vi "NI 9260 Generate Signal (Host).vi"() -> ()   [LabVIEW 2021]
uses:
  <vilib>/LabVIEW Targets/FPGA/cRIO/shared/nicrio_ModuleControls/nicrio_cRIO-9260_DataRatesRing2.ctl
  <vilib>/FPGAPlugInAG/cRIO-9053/niLvFpga_Open_cRIO-9053.vi
  <vilib>/rvi/interface/common/dynamic/niFpgaDynamicAddResources.vi
  <vilib>/Utility/error.llb/Error Cluster From Error Code.vi
  <vilib>/rvi/errors/niLvFpgaAdjustHostInterfaceError.vi
  <vilib>/rvi/interface/common/niFpgaWaitOnOcc.vi
  <vilib>/FPGAPlugInAG/Dynamic/niLvFpga_Run_Dynamic.vi
  <vilib>/FPGAPlugInAG/Dynamic/niLvFpga_Close_Dynamic.vi
  <vilib>/rvi/interface/nirviOpenFPGA/nirviOpenFPGA.xnode
  FPGA Bitfiles/crio-ni9260_FPGATarget_NI9260GenerateSi_CtzEkzqCx3U.lvbitx
  NI 9260 Generate Signal (FPGA).vi
  <vilib>/rvi/interface/nirviReadWriteControl/nirviReadWriteControl.xnode
  <vilib>/rvi/interface/nirviMethod/nirviMethod.xnode
  <vilib>/rvi/interface/nirviCloseFPGA/nirviCloseFPGA.xnode
  <vilib>/rvi/interface/Simulation/niFpgaSimulationCallBeginRW.vi
  <vilib>/FPGAPlugInAG/Dynamic/niLvFpga_WriteFifo_Dynamic.vi
  <vilib>/rvi/errors/niLvFpgaMergeErrorWithErrorCode.vi
  NiFpgaLv.dll
  <vilib>/FPGAPlugInAG/Dynamic/niLvFpga_ConfigureFifo_Dynamic.vi
panel:
  out "loop time (ms)":u32
  in  "Waveform":T1(ring)=enum."Square Wave"
  in  "Host Loop Rate (ms)":u32=100
  out "FIFO Time Out":bool
  out "Overvoltage":bool[](array[boolean])
  out "Underflow":bool[](array[boolean])
  in  "Sine Waveform Settings":T2(array[cluster])=[{"Frequency (Hz)"=1000.0, "Amplitude (V)"=4.0, "Offset (V)"=0.0, "Phase (deg)"=0.0}, {"Frequency (Hz)"=100.0, "Amplitude (V)"=3.0, "Offset (V)"=0.0, "Phase (deg)"=0.0}]
  in  "stop":bool
  out "FPGA Error out":errorcluster
  in  "Number of Samples per channel":dbl=51200.0 format="%.2p"
  out "Analog Output":waveform(dbl)[](graph)
  in  "Data Rate":T3=1 items=["51.200 kS/s (NI 9260)"=1, "25.600 kS/s (NI 9260)"=2, "17.067 kS/s (NI 9260)"=3, "12.800 kS/s (NI 9260)"=4, "10.240 kS/s (NI 9260)"=5, "8.533 kS/s (NI 9260)"=6, "7.314 kS/s (NI 9260)"=7, "6.400 kS/s (NI 9260)"=8, "5.689 kS/s (NI 9260)"=9, "5.120 kS/s (NI 9260)"=10, "4.654 kS/s (NI 9260)"=11, "4.267 kS/s (NI 9260)"=12, "3.938 kS/s (NI 9260)"=13, "3.657 kS/s (NI 9260)"=14, "3.413 kS/s (NI 9260)"=15, "3.200 kS/s (NI 9260)"=16, "3.012 kS/s (NI 9260)"=17, "2.845 kS/s (NI 9260)"=18, "2.695 kS/s (NI 9260)"=19, "2.560 kS/s (NI 9260)"=20, "2.438 kS/s (NI 9260)"=21, "2.328 kS/s (NI 9260)"=22, "2.226 kS/s (NI 9260)"=23, "2.133 kS/s (NI 9260)"=24, "2.048 kS/s (NI 9260)"=25, "1.969 kS/s (NI 9260)"=26, "1.896 kS/s (NI 9260)"=27, "1.829 kS/s (NI 9260)"=28, "1.765 kS/s (NI 9260)"=29, "1.707 kS/s (NI 9260)"=30, "1.652 kS/s (NI 9260)"=31]
  out "Host Error out":errorcluster
  # "Overview: Demonstrates how to generate a sine wave from the NI 9260\nRequirements: LabVIEW Full Development System, LV FPGA, and NI RIO\nInstructions: \n1. The NI 9260 will drive its outputs to 0 volts when the module receives a start command. Some DUTs will be affected by the sudden drop to zero from the previous value seen at the output. See the  NI 9260 Advanced example for how to mitigate this behavior.  \n2. Run this VI."
  # "CH0"
  # "CH1"
  # "CH0"
  # "CH1"
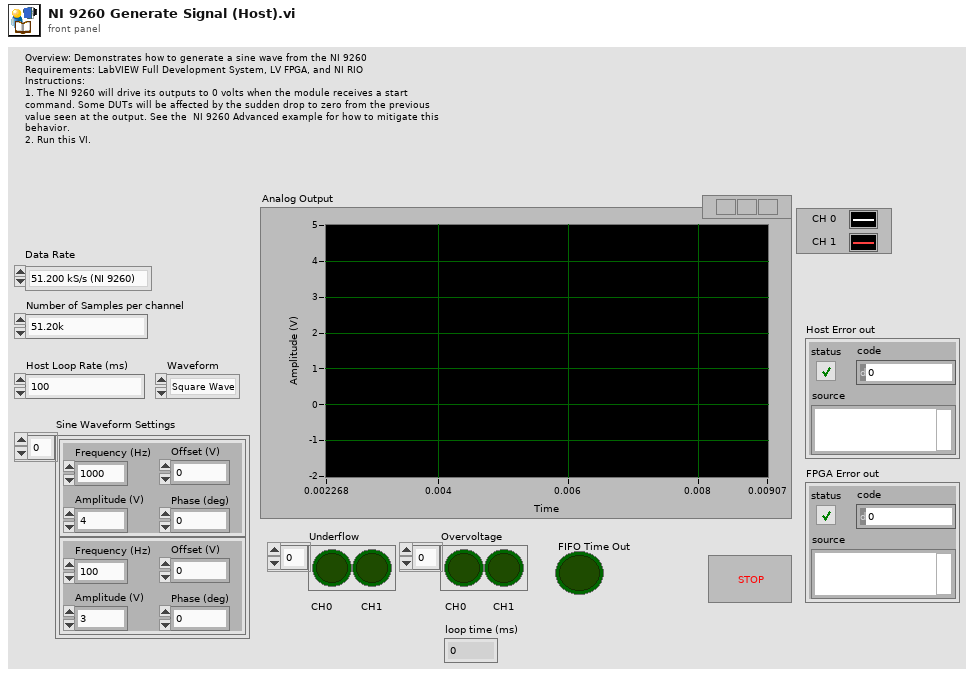
[diagram p1: front panel]
types:
  T1 = enum16{"Sawtooth Wave", "Square Wave", "Sine Wave"}
  T2 = cluster{"Frequency (Hz)":dbl, "Amplitude (V)":dbl, "Offset (V)":dbl, "Phase (deg)":dbl}[]
  T3 = typedef "nicrio_cRIO-9260_DataRatesRing2.ctl" = u8
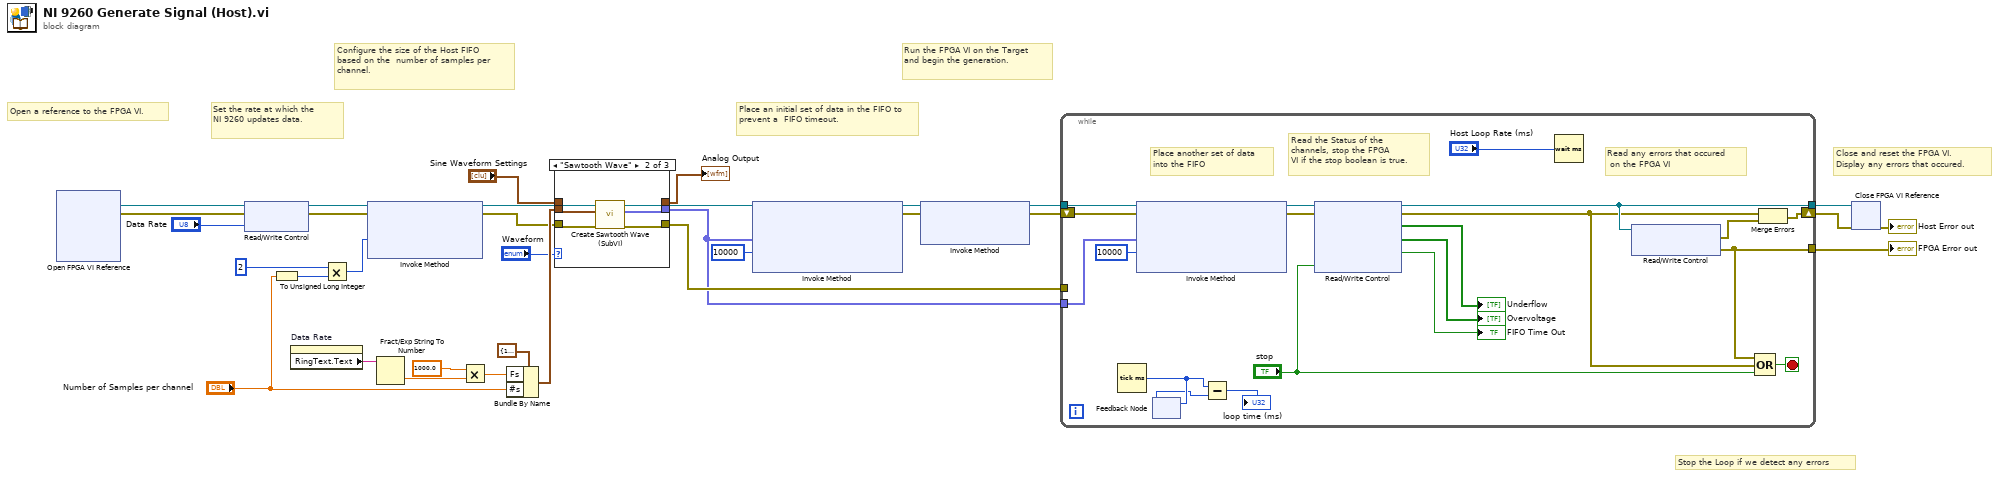
[diagram p0: block diagram]
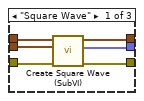
[diagram p2: hidden frame]
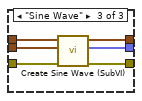
[diagram p3: hidden frame]
diagram:
  # "Place an initial set of data in the FIFO to prevent a  FIFO timeout."
  # "Stop the Loop if we detect any errors"
  # "Configure the size of the Host FIFO based on the  number of samples per channel."
  # "Set the rate at which the \nNI 9260 updates data."
  # "Close and reset the FPGA VI. \nDisplay any errors that occured."
  # "Run the FPGA VI on the Target and begin the generation."
  # "Open a reference to the FPGA VI."
  n1 = xnode "Open FPGA VI Reference"() -> ("FPGA VI Reference Out"=w29:refnum<k20>, "error out"=w31:errorcluster)  [unwired: 2 in]
  n2 = xnode "Read/Write Control"("FPGA VI Reference In"=w29, "error in"=w31, "Data Rate"="Data Rate") -> ("FPGA VI Reference Out"=w23:refnum<k20>, "error out"=w14:errorcluster)
  n3 = To Unsigned Long Integer(number="Number of Samples per channel") -> (unsigned 32bit integer=w20:u32)
  n4 = property on="Data Rate" class="Ring (strict)"() -> ("RingText.Text"=w26:string)  [unwired: 2 in, 2 out]
  n5 = Multiply(x=u32 2, y=w20) -> (x*y=w22:u32)
  n6 = xnode "Invoke Method"("FPGA VI Reference In"=w23, "error in"=w14, "Requested Depth"=w22) -> ("FPGA VI Reference Out"=w16:refnum<k20>, "error out"=w5:errorcluster)  [unwired: 1 out]
  n7 = Fract/Exp String To Number(string=w26) -> (number=w25:dbl)  [unwired: 3 in, 1 out]
  n8 = Multiply(x=1000.0, y=w25) -> (x*y=w11:dbl)
  n9 = Bundle By Name(cluster=cluster{"Fs":dbl, "#s":dbl} {"Fs"=1000.0, "#s"=1000.0} ("sampling info"), "Fs"=w11, "#s"="Number of Samples per channel") -> (w6:cluster{"Fs":dbl, "#s":dbl})
  n10 = case shown="\"Sawtooth Wave\"" "Waveform" {
    tunnel: w5 -> [w35 w41 w49]
    tunnel: "Sine Waveform Settings" -> [w37 w43 w48]
    tunnel: w6 -> [w36 w42 w47]
    tunnel: [w32 w38 w46] -> w1
    tunnel: [w34 w39 w45] -> w4
    tunnel: [w33 w40 w44] -> w3
    frame "Square Wave" {
      n11 = call "Create Square Wave (SubVI).vi"("error in (no error)"=w35, "sampling info"=w36, "Sine Waveform Settings"=w37) -> ("error out"=w34:errorcluster, "FXP Sinewave"=w32:fxp<+/-,24,4>[], "Voltage Output Waveform"=w33:waveform(dbl)[])  [unwired: 6 in]
    }
    frame "Sawtooth Wave" {
      n12 = call "Create Sawtooth Wave (SubVI).vi"("error in (no error)"=w41, "sampling info"=w42, "Sine Waveform Settings"=w43) -> ("error out"=w39:errorcluster, "FXP Sinewave"=w38:fxp<+/-,24,4>[], "Voltage Output Waveform"=w40:waveform(dbl)[])  [unwired: 6 in]
    }
    frame "Sine Wave" {
      n13 = call "Create Sine Wave (SubVI).vi"("error in (no error)"=w49, "sampling info"=w47, "Sine Waveform Settings"=w48) -> ("error out"=w45:errorcluster, "FXP Sinewave"=w46:fxp<+/-,24,4>[], "Voltage Output Waveform"=w44:waveform(dbl)[])  [unwired: 6 in]
    }
  }
  "Analog Output" <- w3
  n14 = xnode "Invoke Method"("FPGA VI Reference In"=w16, "Data"=w1, "Timeout (ms)"=10000) -> ("FPGA VI Reference Out"=w15:refnum<k20>, "error out"=w17:errorcluster)  [unwired: 1 in, 1 out]
  n15 = xnode "Invoke Method"("FPGA VI Reference In"=w15, "error in"=w17) -> ("FPGA VI Reference Out"=w18:refnum<k20>, "error out"=w19:errorcluster)  [unwired: 1 in]
  n16 = while {
    tunnel: w18 -> [w67]
    tunnel: w4 -> [_]
    tunnel: [w58] -> w12
    tunnel: [w56] -> w8
    shift-right: [w55] -> w24
    shift-left: w19 -> [w65]
    tunnel: w1 -> [w53]
    stop <- w64 stop-if-true
    # "Read any errors that occured\n on the FPGA VI"
    # "Read the Status of the \nchannels, stop the FPGA \nVI if the stop boolean is true."
    # "Place another set of data\ninto the FIFO"
    n17 = Tick Count (ms)() -> (millisecond timer value=w52:u32)
    n18 = xnode "Invoke Method"("FPGA VI Reference In"=w67, "error in"=w65, "Data"=w53, "Timeout (ms)"=10000) -> ("FPGA VI Reference Out"=w69:refnum<k20>, "error out"=w68:errorcluster)  [unwired: 1 out]
    n19 = feedback-in #1(w52) -> ()
    n20 = feedback #1() -> (w51:u32)  [unwired: 1 in]
    n21 = Subtract(x=w52, y=w51) -> (x-y=→"loop time (ms)":u32)
    n22 = xnode "Read/Write Control"("FPGA VI Reference In"=w69, "error in"=w68, "stop"="stop") -> ("FPGA VI Reference Out"=w58:refnum<k20>, "error out"=w57:errorcluster, "Underflow"=→"Underflow":bool[], "Overvoltage"=→"Overvoltage":bool[], "FIFO Time Out"=→"FIFO Time Out":bool)
    n23 = Wait (ms)(milliseconds to wait="Host Loop Rate (ms)") -> ()  [unwired: 1 out]
    n24 = xnode "Read/Write Control"("FPGA VI Reference In"=w58) -> ("error out"=w54:errorcluster, "FPGA Error out"=w56:errorcluster)  [unwired: 1 in, 1 out]
    n25 = Compound Arithmetic op=OR(w56, w57, "stop") -> (w64:bool)
    n26 = Merge Errors(w57, w54) -> (w55:errorcluster)
  }
  "FPGA Error out" <- w8
  n27 = xnode "Close FPGA VI Reference"("FPGA VI Reference In"=w12, "error in"=w24) -> ("error out"=→"Host Error out":errorcluster)
